vi "PI_GCS2_All_VIs.vi"   [LabVIEW 2026]
doc: "This VI contains all high level and low level VIs valid for PI GCS2 devices. \nSee diagram for a survey of all PI GCS2 high level and low level VIs. \nMenu / Browse / Show VI Hierarchy will show the file paths of the VIs. \nGlobal Variables are shown as Control as well as Indicator."
uses:
  Low Level/Communication/Global1.vi
  Low Level/GeneralCommands/Controller names.ctl
  Low Level/Communication/Available DLL interfaces.ctl
  Low Level/Communication/Available DLLs.ctl
  Low Level/Communication/Available interfaces.ctl
  Low Level/Communication/Termination character.ctl
  Low Level/GeneralCommands/Global2 (Array).vi
  Low Level/Communication/Global DaisyChain.vi
  Low Level/Support/HasCommandArray.vi
  Low Level/Support/GCSArray_regex_selector.ctl
  Low Level/Communication/Syntax.ctl
  Low Level/GeneralCommands/CommandInfo.ctl
  Low Level/GeneralCommands/MemoryType.ctl
  Low Level/GeneralCommands/Parameter Set.ctl
  Low Level/GeneralCommands/ParameterInfoSet.ctl
  Low Level/GeneralCommands/UnitDescription.ctl
  Low Level/SpecialCommand/UserCommandLevel.ctl
  Low Level/Communication/Configuration Setup State.ctl
  Low Level/GeneralCommands/HardwareInfo.ctl
  Low Level/GeneralCommands/DynamicHardwareInfo.ctl
  Low Level/GeneralCommands/FirmwareInfo.ctl
  Low Level/SpecialCommand/RecorderStatus.ctl
  Low Level/SpecialCommand/RecorderTraceConfiguration.ctl
  Low Level/SpecialCommand/RecorderTriggerConfiguration.ctl
  Low Level/SpecialCommand/DriveStateMachine.ctl
  Low Level/SpecialCommand/ModeOfOperation.ctl
  Low Level/GeneralCommands/AxisStatus.ctl
  Low Level/GeneralCommands/SystemStatus.ctl
  Low Level/GeneralCommands/Status.ctl
panel:
  # "PI GCS2 LabVIEW driver set"
  # "This VI contains all high level and low level VIs valid for PI GCS2 devices. See diagram for a survey of all PI GCS2 high level and low level VIs. Menu / Browse / Show VI Hierarchy will show the file paths of the VIs. Global Variables are shown as Control as well as Indicator."
types:
  T1 = typedef "Status.ctl" = cluster{"Element":string, "Status bits":bool[]}
  T2 = typedef "SystemStatus.ctl" = cluster{"Element":string, "Command Error":bool, "Critical Error":bool, "Information":bool, "Warning":bool}
  T3 = typedef "AxisStatus.ctl" = cluster{"Element":string, "Error":bool, "EAX?":bool, "Drive State Machine":T4, "Mode of Operation":T5, "OL/CL control active?":bool, "ONT?":bool, "In Motion":bool, "FRF?":bool, "IPR":bool, "Plim":bool, "Nlim":bool}
  T4 = typedef "DriveStateMachine.ctl" = u16
  T5 = typedef "ModeOfOperation.ctl" = enum16{"Open", "Open-Loop Position", "Closed-Loop Position", "Open-Loop Velocity", "Closed-Loop Velocity", "Open-Loop Force", "Closed-Loop Force", "Step Operation"}
  T6 = typedef "RecorderTriggerConfiguration.ctl" = cluster{"RecorderID":string, "RecorderTrigger":string, "AxisID":string, "Recurring":string}
  T7 = typedef "RecorderTraceConfiguration.ctl" = cluster{"RecorderID":string, "TraceID":i32, "Container Unit":string, "Function Unit":string, "ParameterID":i32}
  T8 = typedef "RecorderStatus.ctl" = enum16{"RUN", "CFG", "WAIT"}
  T9 = typedef "FirmwareInfo.ctl" = cluster{"Container Unit":string, "Function Unit":string, "ID":string, "Mathccode":string, "Version":string, "Date":string, "Compatibility":string, "Description":string}
  T10 = typedef "DynamicHardwareInfo.ctl" = cluster{"Property":string, "Type":string, "Value":string}
  T11 = typedef "HardwareInfo.ctl" = cluster{"Matchcode":string, "Version":string, "Serial Number":string, "Date":string, "Dynamic Hardware":cluster{"Property":string, "Type":string, "Value":string}[], "Firmware":cluster{"Container Unit":string, "Function Unit":string, "ID":string, "Mathccode":string, "Version":string, "Date":string, "Compatibility":string, "Description":string}[]}
  T12 = typedef "Configuration Setup State.ctl" = enum16{"Do nothing", "Initialize indicators", "Select Connection", "TCP/IP Connection", "RS232 Connection", "USB Connection", "Board Connection", "DaisyChain Connection", "Open Interface", "Read IDs", "Prepare referencing", "Reference", "Servo", "Query Status", "Misc", "WaveGenerator", "Control Mode", "Enable Axes", "Translate Error", "Hexapod", "Piezo"}
  T13 = typedef "UserCommandLevel.ctl" = enum16{"User", "Expert", "PI Staff", "FW Developer"}
  T14 = typedef "UnitDescription.ctl" = cluster{"Container Unit":string, "Function Unit":string, "Description":string}
  T15 = typedef "ParameterInfoSet.ctl" = cluster{"Container Unit":string, "Function Unit":string, "Parameter ID":string, "DataType":string, "Dimension":string, "Read UCL":string, "Write UCL":string, "Min Value":string, "Max Value":string, "Parameter Type":string, "Description":string}
  T16 = typedef "Parameter Set.ctl" = cluster{"Memory Type":T17, "Container Unit":string, "Function Unit":string, "Parameter ID":string, "Parameter Value":string}
  T17 = typedef "MemoryType.ctl" = enum16{"<No Setting>", "RAM", "FLASH", "TMP"}
  T18 = typedef "CommandInfo.ctl" = cluster{"Command":string, "Command Signatur":string, "Description":string}
  T19 = typedef "GCSArray_regex_selector.ctl" = enum16{"GCS_ARRAY Block Full", "GCS_ARRAY Block ID", "GCS_ARRAY Block Header", "GCS_ARRAY Block Data", "GCS_ARRAY Identifier", "GCS_ARRAY Remark", "GCS_ARRAY Version", "GCS_ARRAY Dimension", "GCS_ARRAY Type", "GCS_ARRAY Separator", "GCS_ARRAY NData", "GCS_ARRAY NData%", "GCS_ARRAY NData% Keyword", "GCS_ARRAY Name%", "GCS_ARRAY Name% Keyword", "GCS_ARRAY Start%", "GCS_ARRAY Start% Keyword", "GCS_ARRAY End%", "GCS_ARRAY End% Keyword", "GCS_ARRAY Delta%", "GCS_ARRAY Delta% Keword", "GCS_ARRAY Sample Time", "GCS_ARRAY Unit of transmitted value%", "GCS_ARRAY Trans_Unit% Keyword", "GCS_ARRAY Trans_Unit% = RAW Keyword", "GCS_ARRAY Unit of displayed value%", "GCS_ARRAY Disp_Unit% Keyword", "GCS_ARRAY Nominator%", "GCS_ARRAY Ratio_Nom% Keyword", "GCS_ARRAY Denominator%", "GCS_ARRAY Ratio_Denom% Keyword", "GCS_ARRAY End of Header", "GCS_ARRAY Empty line of Header"}
  T20 = typedef "Syntax.ctl" = enum16{"GCS 1.0", "GCS 2.0", "GCS 3.0"}
  T21 = typedef "Termination character.ctl" = enum16{"LF", "CR", "LFCR", "CRLF"}
  T22 = typedef "Available interfaces.ctl" = u16
  T23 = typedef "Available DLLs.ctl" = u16
  T24 = typedef "Available DLL interfaces.ctl" = u16
  T25 = typedef "Controller names.ctl" = enum16{"None", "Analog", "C-702", "C-413", "C-414", "C-843", "C-843.PM", "C-844", "C-848", "C-865", "C-866", "C-867", "C-877", "C-880", "C-884", "C-885", "C-886", "C-887", "C-891", "E-135", "E-516", "E-517", "E-518", "E-709", "E-710", "E-712", "E-725", "E-727", "E-753", "E-754", "E-755", "E-761", "E-816", "E-861", "E-870", "E-871", "E-872", "E-873", "E-874", "F-206", "HydraPollux", "M-840", "M-850", "M-8X0", "Mercury", "Mercury_GCS", "PI_GCS2"}
  T26 = cluster{"No. of devices":i32, "Port ID":i32, "Devices":string[], "Description":string}[]
  T27 = cluster{"Conn. axes":string[], "Controller name":T25}[]
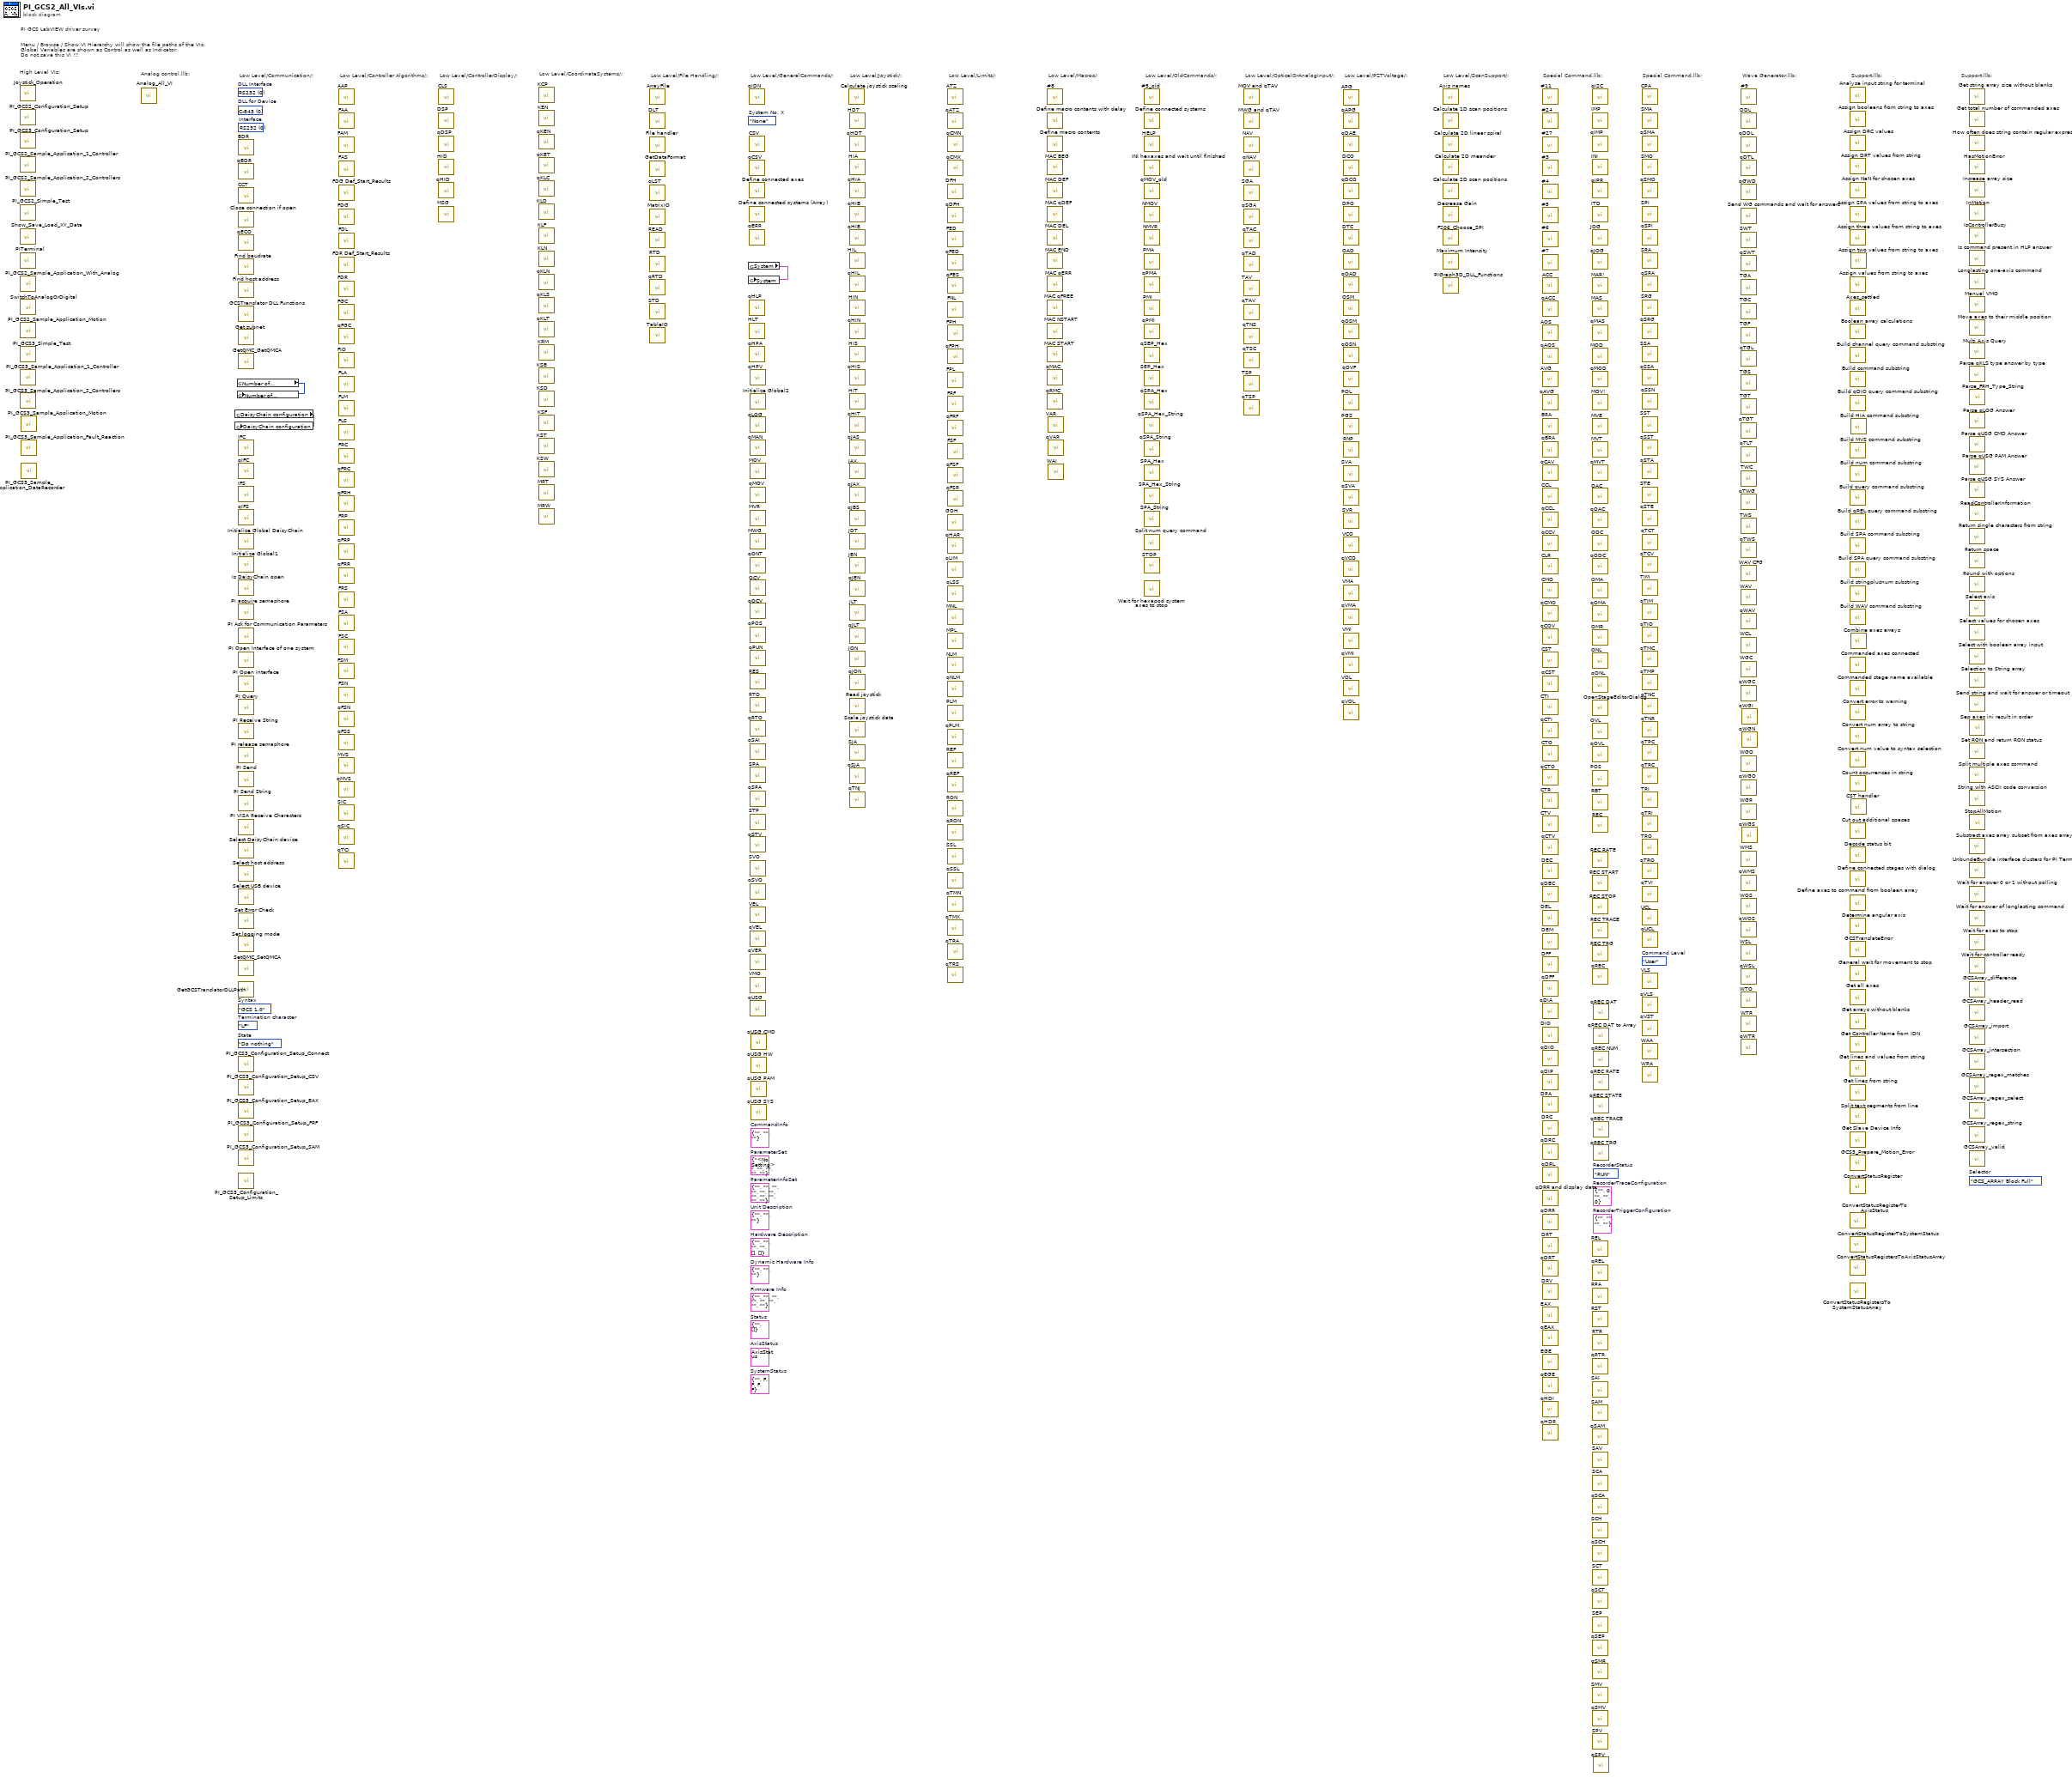
[diagram p0: block diagram]
diagram:
  (unwired) T1 {"Element"="", "Status bits"=[]}  # Status
  (unwired) T2 {"Element"="", "Command Error"=FALSE, "Critical Error"=FALSE, "Information"=FALSE, "Warning"=FALSE}  # SystemStatus
  (unwired) T3 {"Element"="", "Error"=FALSE, "EAX?"=FALSE, "Drive State Machine"=0, "Mode of Operation"=enum."Open", "OL/CL control active?"=FALSE, "ONT?"=FALSE, "In Motion"=FALSE, "FRF?"=FALSE, "IPR"=FALSE, "Plim"=FALSE, "Nlim"=FALSE}  # AxisStatus
  (unwired) T6 {"RecorderID"="", "RecorderTrigger"="", "AxisID"="", "Recurring"=""}  # RecorderTriggerConfiguration
  (unwired) T7 {"RecorderID"="", "TraceID"=0, "Container Unit"="", "Function Unit"="", "ParameterID"=0}  # RecorderTraceConfiguration
  (unwired) RecorderStatus."RUN"  # RecorderStatus
  (unwired) T9 {"Container Unit"="", "Function Unit"="", "ID"="", "Mathccode"="", "Version"="", "Date"="", "Compatibility"="", "Description"=""}  # Firmware Info
  (unwired) T10 {"Property"="", "Type"="", "Value"=""}  # Dynamic Hardware Info
  (unwired) T11 {"Matchcode"="", "Version"="", "Serial Number"="", "Date"="", "Dynamic Hardware"=[], "Firmware"=[]}  # Hardware Description
  (unwired) Configuration_Setup_State."Do nothing"  # State
  (unwired) UserCommandLevel."User"  # Command Level
  (unwired) T14 {"Container Unit"="", "Function Unit"="", "Description"=""}  # Unit Description
  (unwired) T15 {"Container Unit"="", "Function Unit"="", "Parameter ID"="", "DataType"="", "Dimension"="", "Read UCL"="", "Write UCL"="", "Min Value"="", "Max Value"="", "Parameter Type"="", "Description"=""}  # ParameterInfoSet
  (unwired) T16 {"Memory Type"=enum."<No Setting>", "Container Unit"="", "Function Unit"="", "Parameter ID"="", "Parameter Value"=""}  # ParameterSet
  (unwired) T18 {"Command"="", "Command Signatur"="", "Description"=""}  # CommandInfo
  (unwired) GCSArray_regex_selector."GCS_ARRAY Block Full"  # Selector
  (unwired) Syntax."GCS 1.0"  # Syntax
  (unwired) Termination_character."LF"  # Termination character
  (unwired) T22 0 items=["RS232", "GPIB", "DLL", "TCP-IP"]  # Interface
  (unwired) T23 0 items=["C-843", "C-844", "E-710", "C-843.PM", "C-865", "E-761", "Mercury", "E-755", "E-753", "C-866", "E-712", "E-725", "E-861", "C-867", "E-517", "E-816", "E-709", "PI_GCS2_DLL"]  # DLL for Device
  (unwired) T24 0 items=["RS232", "GPIB", "Board", "TCP-IP", "USB", "RS232_DC", "USB_DC"]  # DLL Interface
  (unwired) Controller_names."None"  # System No. X
  # "Low Level/CoordinateSystems/:"
  # "High Level VIs:"
  # "Analog control.llb:"
  # "Support.llb:"
  # "Wave Generator.llb:"
  # "Special Command.llb:"
  # "Support.llb:"
  # "Special Command.llb:"
  # "Low Level/ScanSupport/:"
  # "Low Level/PZTVoltage/:"
  # "Low Level/OpticalOrAnalogInput/:"
  # "Low Level/OldCommands/:"
  # "Low Level/Macros/:"
  # "Low Level/Limits/:"
  # "Low Level/Joystick/:"
  # "Low Level/GeneralCommands/:"
  # "Low Level/File Handling/:"
  # "Low Level/ControllerDisplay/:"
  # "Low Level/Controller Algorithms/:"
  # "Menu / Browse / Show VI Hierarchy will show the file paths of the VIs. \nGlobal Variables are shown as Control as well as Indicator.\nDo not save this VI !!!"
  # "PI GCS LabVIEW driver survey"
  # "Low Level/Communication/:"
  n1 = call "Joystick_Operation.vi"() -> ()  [unwired: 15 in, 5 out]
  n2 = call "PI_GCS2_Configuration_Setup.vi"() -> ()  [unwired: 8 in, 12 out]
  n3 = call "PI_GCS3_Configuration_Setup.vi"() -> ()  [unwired: 14 in, 6 out]
  n4 = call "PI_GCS2_Sample_Application_1_Controller.vi"() -> ()  [unwired: 1 out]
  n5 = call "PI_GCS2_Sample_Application_2_Controllers.vi"() -> ()  [unwired: 1 out]
  n6 = call "PI_GCS2_Simple_Test.vi"() -> ()  [unwired: 20 out]
  n7 = call "Show_Save_Load_XY_Data.vi"() -> ()  [unwired: 7 in, 13 out]
  n8 = call "PITerminal.vi"() -> ()  [unwired: 2 in, 18 out]
  n9 = call "PI_GCS2_Sample_Application_With_Analog.vi"() -> ()  [unwired: 1 out]
  n10 = call "SwitchToAnalogOrDigital.vi"() -> ()  [unwired: 9 in, 11 out]
  n11 = call "PI_GCS2_Sample_Application_Motion.vi"() -> ()  [unwired: 1 in]
  n12 = call "PI_GCS3_Simple_Test.vi"() -> ()  [unwired: 20 in]
  n13 = call "PI_GCS3_Sample_Application_1_Controller.vi"() -> ()  [unwired: 1 in]
  n14 = call "PI_GCS3_Sample_Application_2_Controllers.vi"() -> ()  [unwired: 1 in]
  n15 = call "PI_GCS3_Sample_Application_Motion.vi"() -> ()  [unwired: 1 in]
  n16 = call "PI_GCS3_Sample_Application_Fault_Reaction.vi"() -> ()  [unwired: 20 in]
  n17 = call "PI_GCS3_Sample_Application_DataRecorder.vi"() -> ()  [unwired: 20 in]
  n18 = call "Analog_All_VI.vi"() -> ()  [unwired: 12 out]
  n19 = global read "Global DaisyChain.vi" "DaisyChain configuration"() -> (w1:T26)
  n20 = global write "Global DaisyChain.vi" "DaisyChain configuration"(w1) -> ()
  n21 = global read "Global1.vi" "Number of\nsystems"() -> (w3:i32)
  n22 = global write "Global1.vi" "Number of\nsystems"(w3) -> ()
  n23 = call "BDR.vi"() -> ()  [unwired: 4 in, 16 out]
  n24 = call "qBDR.vi"() -> ()  [unwired: 2 in, 18 out]
  n25 = call "CCT.vi"() -> ()  [unwired: 3 in, 17 out]
  n26 = call "Close connection if open.vi"() -> ()  [unwired: 3 in, 17 out]
  n27 = call "qECO.vi"() -> ()  [unwired: 3 in, 17 out]
  n28 = call "Find baudrate.vi"() -> ()  [unwired: 10 in, 10 out]
  n29 = call "Find host address.vi"() -> ()  [unwired: 6 in, 14 out]
  n30 = call "GCSTranslator DLL Functions.vi"() -> ()  [unwired: 7 in, 13 out]
  n31 = call "Get subnet.vi"() -> ()  [unwired: 20 out]
  n32 = call "GetQMC_GetQMCA.vi"() -> ()  [unwired: 6 in, 14 out]
  n33 = call "IFC.vi"() -> ()  [unwired: 4 in, 16 out]
  n34 = call "qIFC.vi"() -> ()  [unwired: 4 in, 16 out]
  n35 = call "IFS.vi"() -> ()  [unwired: 5 in, 15 out]
  n36 = call "qIFS.vi"() -> ()  [unwired: 4 in, 16 out]
  n37 = call "Initialize Global DaisyChain.vi"() -> ()  [unwired: 2 in, 18 out]
  n38 = call "Initialize Global1.vi"() -> ()  [unwired: 2 in, 18 out]
  n39 = call "Is DaisyChain open.vi"() -> ()  [unwired: 2 in, 18 out]
  n40 = call "PI acquire semaphore.vi"() -> ()  [unwired: 2 in, 18 out]
  n41 = call "PI Ask for Communication Parameters.vi"() -> ()  [unwired: 20 out]
  n42 = call "PI Open Interface of one system.vi"() -> ()  [unwired: 12 in, 8 out]
  n43 = call "PI Open Interface.vi"() -> ()  [unwired: 12 in, 8 out]
  n44 = call "PI Query.vi"() -> ()  [unwired: 7 in, 13 out]
  n45 = call "PI Receive String.vi"() -> ()  [unwired: 3 in, 17 out]
  n46 = call "PI release semaphore.vi"() -> ()  [unwired: 4 in, 16 out]
  n47 = call "PI Send.vi"() -> ()  [unwired: 6 in, 14 out]
  n48 = call "PI Send String.vi"() -> ()  [unwired: 4 in, 16 out]
  n49 = call "PI VISA Receive Characters.vi"() -> ()  [unwired: 3 in, 17 out]
  n50 = call "Select DaisyChain device.vi"() -> ()  [unwired: 9 in, 11 out]
  n51 = call "Select host address.vi"() -> ()  [unwired: 6 in, 14 out]
  n52 = call "Select USB device.vi"() -> ()  [unwired: 5 in, 15 out]
  n53 = call "Set Error Check.vi"() -> ()  [unwired: 2 in, 10 out]
  n54 = call "Set logging mode.vi"() -> ()  [unwired: 4 in, 16 out]
  n55 = call "SetQMC_SetQMCA.vi"() -> ()  [unwired: 8 in, 12 out]
  n56 = call "GetGCSTranslatorDLLPath.vi"() -> ()  [unwired: 1 in, 1 out]
  n57 = call "PI_GCS3_Configuration_Setup_Connect.vi"() -> ()  [unwired: 19 in, 1 out]
  n58 = call "PI_GCS3_Configuration_Setup_CSV.vi"() -> ()  [unwired: 19 in, 1 out]
  n59 = call "PI_GCS3_Configuration_Setup_EAX.vi"() -> ()  [unwired: 19 in, 1 out]
  n60 = call "PI_GCS3_Configuration_Setup_FRF.vi"() -> ()  [unwired: 19 in, 1 out]
  n61 = call "PI_GCS3_Configuration_Setup_SAM.vi"() -> ()  [unwired: 19 in, 1 out]
  n62 = call "PI_GCS3_Configuration_Setup_Limits.vi"() -> ()  [unwired: 17 in, 3 out]
  n63 = call "AAP.vi"() -> ()  [unwired: 12 in, 8 out]
  n64 = call "FAA.vi"() -> ()  [unwired: 11 in, 9 out]
  n65 = call "FAM.vi"() -> ()  [unwired: 11 in, 9 out]
  n66 = call "FAS.vi"() -> ()  [unwired: 11 in, 9 out]
  n67 = call "FDG Def_Start_Results.vi"() -> ()  [unwired: 12 in, 8 out]
  n68 = call "FDG.vi"() -> ()  [unwired: 12 in, 8 out]
  n69 = call "FDL.vi"() -> ()  [unwired: 19 in, 1 out]
  n70 = call "FDR Def_Start_Results.vi"() -> ()  [unwired: 12 in, 8 out]
  n71 = call "FDR.vi"() -> ()  [unwired: 14 in, 6 out]
  n72 = call "FGC.vi"() -> ()  [unwired: 7 in, 13 out]
  n73 = call "qFGC.vi"() -> ()  [unwired: 4 in, 16 out]
  n74 = call "FIO.vi"() -> ()  [unwired: 13 in, 7 out]
  n75 = call "FLA.vi"() -> ()  [unwired: 13 in, 7 out]
  n76 = call "FLM.vi"() -> ()  [unwired: 13 in, 7 out]
  n77 = call "FLS.vi"() -> ()  [unwired: 13 in, 7 out]
  n78 = call "FRC.vi"() -> ()  [unwired: 5 in, 15 out]
  n79 = call "qFRC.vi"() -> ()  [unwired: 4 in, 16 out]
  n80 = call "qFRH.vi"() -> ()  [unwired: 2 in, 18 out]
  n81 = call "FRP.vi"() -> ()  [unwired: 4 in, 16 out]
  n82 = call "qFRP.vi"() -> ()  [unwired: 4 in, 16 out]
  n83 = call "qFRR.vi"() -> ()  [unwired: 6 in, 14 out]
  n84 = call "FRS.vi"() -> ()  [unwired: 3 in, 17 out]
  n85 = call "FSA.vi"() -> ()  [unwired: 13 in, 7 out]
  n86 = call "FSC.vi"() -> ()  [unwired: 12 in, 8 out]
  n87 = call "FSM.vi"() -> ()  [unwired: 12 in, 8 out]
  n88 = call "FSN.vi"() -> ()  [unwired: 13 in, 7 out]
  n89 = call "qFSN.vi"() -> ()  [unwired: 3 in, 17 out]
  n90 = call "qFSS.vi"() -> ()  [unwired: 2 in, 18 out]
  n91 = call "MVS.vi"() -> ()  [unwired: 8 in, 12 out]
  n92 = call "qMVS.vi"() -> ()  [unwired: 5 in, 15 out]
  n93 = call "SIC.vi"() -> ()  [unwired: 6 in, 14 out]
  n94 = call "qSIC.vi"() -> ()  [unwired: 4 in, 16 out]
  n95 = call "qTCI.vi"() -> ()  [unwired: 3 in, 17 out]
  n96 = call "CLS.vi"() -> ()  [unwired: 2 in, 18 out]
  n97 = call "DSP.vi"() -> ()  [unwired: 5 in, 15 out]
  n98 = call "qDSP.vi"() -> ()  [unwired: 3 in, 17 out]
  n99 = call "HID.vi"() -> ()  [unwired: 5 in, 15 out]
  n100 = call "qHID.vi"() -> ()  [unwired: 3 in, 17 out]
  n101 = call "MSG.vi"() -> ()  [unwired: 3 in, 17 out]
  n102 = call "KCP.vi"() -> ()  [unwired: 4 in, 16 out]
  n103 = call "KEN.vi"() -> ()  [unwired: 3 in, 17 out]
  n104 = call "qKEN.vi"() -> ()  [unwired: 3 in, 17 out]
  n105 = call "qKET.vi"() -> ()  [unwired: 3 in, 17 out]
  n106 = call "qKLC.vi"() -> ()  [unwired: 6 in, 14 out]
  n107 = call "KLD.vi"() -> ()  [unwired: 6 in, 14 out]
  n108 = call "KLF.vi"() -> ()  [unwired: 3 in, 17 out]
  n109 = call "KLN.vi"() -> ()  [unwired: 4 in, 16 out]
  n110 = call "qKLN.vi"() -> ()  [unwired: 3 in, 17 out]
  n111 = call "qKLS.vi"() -> ()  [unwired: 5 in, 15 out]
  n112 = call "qKLT.vi"() -> ()  [unwired: 4 in, 16 out]
  n113 = call "KRM.vi"() -> ()  [unwired: 3 in, 17 out]
  n114 = call "KSB.vi"() -> ()  [unwired: 6 in, 14 out]
  n115 = call "KSD.vi"() -> ()  [unwired: 6 in, 14 out]
  n116 = call "KSF.vi"() -> ()  [unwired: 3 in, 17 out]
  n117 = call "KST.vi"() -> ()  [unwired: 6 in, 14 out]
  n118 = call "KSW.vi"() -> ()  [unwired: 6 in, 14 out]
  n119 = call "MRT.vi"() -> ()  [unwired: 5 in, 15 out]
  n120 = call "MRW.vi"() -> ()  [unwired: 5 in, 15 out]
  n121 = call "ArrayFile.vi"() -> ()  [unwired: 20 out]
  n122 = call "DLT.vi"() -> ()  [unwired: 3 in, 17 out]
  n123 = call "File handler.vi"() -> ()  [unwired: 6 in, 14 out]
  n124 = call "GetDataFormat.vi"() -> ()  [unwired: 2 in, 18 out]
  n125 = call "qLST.vi"() -> ()  [unwired: 2 in, 18 out]
  n126 = call "MatrixIO.vi"() -> ()  [unwired: 7 in, 13 out]
  n127 = call "READ.vi"() -> ()  [unwired: 3 in, 17 out]
  n128 = call "RTD.vi"() -> ()  [unwired: 5 in, 15 out]
  n129 = call "qRTD.vi"() -> ()  [unwired: 2 in, 18 out]
  n130 = call "STD.vi"() -> ()  [unwired: 5 in, 15 out]
  n131 = call "TableIO.vi"() -> ()  [unwired: 6 in, 14 out]
  n132 = global read "Global2 (Array).vi" "System"() -> (w2:T27)
  n133 = global write "Global2 (Array).vi" "System"(w2) -> ()
  n134 = call "qIDN.vi"() -> ()  [unwired: 2 in, 18 out]
  n135 = call "CSV.vi"() -> ()  [unwired: 3 in, 17 out]
  n136 = call "qCSV.vi"() -> ()  [unwired: 2 in, 18 out]
  n137 = call "Define connected axes.vi"() -> ()  [unwired: 5 in, 15 out]
  n138 = call "Define connected systems (Array).vi"() -> ()  [unwired: 4 in, 16 out]
  n139 = call "qERR.vi"() -> ()  [unwired: 2 in, 18 out]
  n140 = call "qHLP.vi"() -> ()  [unwired: 2 in, 18 out]
  n141 = call "HLT.vi"() -> ()  [unwired: 5 in, 15 out]
  n142 = call "qHPA.vi"() -> ()  [unwired: 2 in, 18 out]
  n143 = call "qHPV.vi"() -> ()  [unwired: 2 in, 18 out]
  n144 = call "Initialize Global2.vi"() -> ()  [unwired: 2 in, 18 out]
  n145 = call "qLOG.vi"() -> ()  [unwired: 18 in, 2 out]
  n146 = call "qMAN.vi"() -> ()  [unwired: 3 in, 17 out]
  n147 = call "MOV.vi"() -> ()  [unwired: 5 in, 15 out]
  n148 = call "qMOV.vi"() -> ()  [unwired: 5 in, 15 out]
  n149 = call "MVR.vi"() -> ()  [unwired: 5 in, 15 out]
  n150 = call "MWG.vi"() -> ()  [unwired: 5 in, 15 out]
  n151 = call "qONT.vi"() -> ()  [unwired: 5 in, 15 out]
  n152 = call "OCV.vi"() -> ()  [unwired: 19 in, 1 out]
  n153 = call "qOCV.vi"() -> ()  [unwired: 18 in, 2 out]
  n154 = call "qPOS.vi"() -> ()  [unwired: 5 in, 15 out]
  n155 = call "qPUN.vi"() -> ()  [unwired: 5 in, 15 out]
  n156 = call "RES.vi"() -> ()  [unwired: 19 in, 1 out]
  n157 = call "RTO.vi"() -> ()  [unwired: 5 in, 15 out]
  n158 = call "qRTO.vi"() -> ()  [unwired: 5 in, 15 out]
  n159 = call "qSAI.vi"() -> ()  [unwired: 5 in, 15 out]
  n160 = call "SPA.vi"() -> ()  [unwired: 10 in, 10 out]
  n161 = call "qSPA.vi"() -> ()  [unwired: 7 in, 13 out]
  n162 = call "STP.vi"() -> ()  [unwired: 2 in, 18 out]
  n163 = call "qSTV.vi"() -> ()  [unwired: 18 in, 2 out]
  n164 = call "SVO.vi"() -> ()  [unwired: 5 in, 15 out]
  n165 = call "qSVO.vi"() -> ()  [unwired: 5 in, 15 out]
  n166 = call "VEL.vi"() -> ()  [unwired: 6 in, 14 out]
  n167 = call "qVEL.vi"() -> ()  [unwired: 5 in, 15 out]
  n168 = call "qVER.vi"() -> ()  [unwired: 2 in, 18 out]
  n169 = call "VMO.vi"() -> ()  [unwired: 5 in, 15 out]
  n170 = call-poly "qUSG.vi"() -> ()  [unwired: 18 in, 2 out]
  n171 = call "qUSG CMD.vi"() -> ()  [unwired: 18 in, 2 out]
  n172 = call "qUSG HW.vi"() -> ()  [unwired: 18 in, 2 out]
  n173 = call "qUSG PAM.vi"() -> ()  [unwired: 18 in, 2 out]
  n174 = call "qUSG SYS.vi"() -> ()  [unwired: 18 in, 2 out]
  n175 = call "Calculate joystick scaling.vi"() -> ()  [unwired: 6 in, 14 out]
  n176 = call "HDT.vi"() -> ()  [unwired: 5 in, 15 out]
  n177 = call "qHDT.vi"() -> ()  [unwired: 5 in, 15 out]
  n178 = call "HIA.vi"() -> ()  [unwired: 6 in, 14 out]
  n179 = call "qHIA.vi"() -> ()  [unwired: 5 in, 15 out]
  n180 = call "qHIB.vi"() -> ()  [unwired: 5 in, 15 out]
  n181 = call "qHIE.vi"() -> ()  [unwired: 5 in, 15 out]
  n182 = call "HIL.vi"() -> ()  [unwired: 5 in, 15 out]
  n183 = call "qHIL.vi"() -> ()  [unwired: 5 in, 15 out]
  n184 = call "HIN.vi"() -> ()  [unwired: 4 in, 16 out]
  n185 = call "qHIN.vi"() -> ()  [unwired: 5 in, 15 out]
  n186 = call "HIS.vi"() -> ()  [unwired: 6 in, 14 out]
  n187 = call "qHIS.vi"() -> ()  [unwired: 6 in, 14 out]
  n188 = call "HIT.vi"() -> ()  [unwired: 5 in, 15 out]
  n189 = call "qHIT.vi"() -> ()  [unwired: 7 in, 13 out]
  n190 = call "qJAS.vi"() -> ()  [unwired: 5 in, 15 out]
  n191 = call "JAX.vi"() -> ()  [unwired: 5 in, 15 out]
  n192 = call "qJAX.vi"() -> ()  [unwired: 5 in, 15 out]
  n193 = call "qJBS.vi"() -> ()  [unwired: 5 in, 15 out]
  n194 = call "JDT.vi"() -> ()  [unwired: 5 in, 15 out]
  n195 = call "JEN.vi"() -> ()  [unwired: 3 in, 17 out]
  n196 = call "qJEN.vi"() -> ()  [unwired: 2 in, 18 out]
  n197 = call "JLT.vi"() -> ()  [unwired: 7 in, 13 out]
  n198 = call "qJLT.vi"() -> ()  [unwired: 7 in, 13 out]
  n199 = call "JON.vi"() -> ()  [unwired: 4 in, 16 out]
  n200 = call "qJON.vi"() -> ()  [unwired: 4 in, 16 out]
  n201 = call "Read joystick.vi"() -> ()  [unwired: 2 in, 18 out]
  n202 = call "Scale joystick data.vi"() -> ()  [unwired: 8 in, 12 out]
  n203 = call "SJA.vi"() -> ()  [unwired: 4 in, 16 out]
  n204 = call "qSJA.vi"() -> ()  [unwired: 3 in, 17 out]
  n205 = call "qTNJ.vi"() -> ()  [unwired: 2 in, 18 out]
  n206 = call "ATZ.vi"() -> ()  [unwired: 6 in, 14 out]
  n207 = call "qATZ.vi"() -> ()  [unwired: 5 in, 15 out]
  n208 = call "DFH.vi"() -> ()  [unwired: 5 in, 15 out]
  n209 = call "qDFH.vi"() -> ()  [unwired: 5 in, 15 out]
  n210 = call "FED.vi"() -> ()  [unwired: 5 in, 15 out]
  n211 = call "qFED.vi"() -> ()  [unwired: 5 in, 15 out]
  n212 = call "qFES.vi"() -> ()  [unwired: 5 in, 15 out]
  n213 = call "FNL.vi"() -> ()  [unwired: 5 in, 15 out]
  n214 = call "FPL.vi"() -> ()  [unwired: 5 in, 15 out]
  n215 = call "FRF.vi"() -> ()  [unwired: 5 in, 15 out]
  n216 = call "qFRF.vi"() -> ()  [unwired: 5 in, 15 out]
  n217 = call "GOH.vi"() -> ()  [unwired: 5 in, 15 out]
  n218 = call "qHAR.vi"() -> ()  [unwired: 5 in, 15 out]
  n219 = call "qLIM.vi"() -> ()  [unwired: 5 in, 15 out]
  n220 = call "qLSS.vi"() -> ()  [unwired: 5 in, 15 out]
  n221 = call "MNL.vi"() -> ()  [unwired: 5 in, 15 out]
  n222 = call "MPL.vi"() -> ()  [unwired: 5 in, 15 out]
  n223 = call "NLM.vi"() -> ()  [unwired: 5 in, 15 out]
  n224 = call "qNLM.vi"() -> ()  [unwired: 5 in, 15 out]
  n225 = call "PLM.vi"() -> ()  [unwired: 5 in, 15 out]
  n226 = call "qPLM.vi"() -> ()  [unwired: 5 in, 15 out]
  n227 = call "REF.vi"() -> ()  [unwired: 5 in, 15 out]
  n228 = call "qREF.vi"() -> ()  [unwired: 5 in, 15 out]
  n229 = call "RON.vi"() -> ()  [unwired: 5 in, 15 out]
  n230 = call "qRON.vi"() -> ()  [unwired: 5 in, 15 out]
  n231 = call "SSL.vi"() -> ()  [unwired: 5 in, 15 out]
  n232 = call "qSSL.vi"() -> ()  [unwired: 5 in, 15 out]
  n233 = call "qTMN.vi"() -> ()  [unwired: 5 in, 15 out]
  n234 = call "qTMX.vi"() -> ()  [unwired: 5 in, 15 out]
  n235 = call "qTRS.vi"() -> ()  [unwired: 5 in, 15 out]
  n236 = call "qCMN.vi"() -> ()  [unwired: 5 in, 15 out]
  n237 = call "qCMX.vi"() -> ()  [unwired: 5 in, 15 out]
  n238 = call "FPH.vi"() -> ()  [unwired: 5 in, 15 out]
  n239 = call "qFPH.vi"() -> ()  [unwired: 5 in, 15 out]
  n240 = call "FSF.vi"() -> ()  [unwired: 8 in, 12 out]
  n241 = call "qFSF.vi"() -> ()  [unwired: 5 in, 15 out]
  n242 = call "qFSR.vi"() -> ()  [unwired: 4 in, 16 out]
  n243 = call "qTRA.vi"() -> ()  [unwired: 5 in, 15 out]
  n244 = call "#8.vi"() -> ()  [unwired: 2 in, 18 out]
  n245 = call "Define macro contents with delay.vi"() -> ()  [unwired: 4 in, 16 out]
  n246 = call "Define macro contents.vi"() -> ()  [unwired: 3 in, 17 out]
  n247 = call "MAC BEG.vi"() -> ()  [unwired: 3 in, 17 out]
  n248 = call "MAC DEF.vi"() -> ()  [unwired: 3 in, 17 out]
  n249 = call "MAC qDEF.vi"() -> ()  [unwired: 2 in, 18 out]
  n250 = call "MAC DEL.vi"() -> ()  [unwired: 4 in, 16 out]
  n251 = call "MAC END.vi"() -> ()  [unwired: 2 in, 18 out]
  n252 = call "MAC qERR.vi"() -> ()  [unwired: 2 in, 18 out]
  n253 = call "MAC qFREE.vi"() -> ()  [unwired: 2 in, 18 out]
  n254 = call "MAC NSTART.vi"() -> ()  [unwired: 5 in, 15 out]
  n255 = call "MAC START.vi"() -> ()  [unwired: 4 in, 16 out]
  n256 = call "qMAC.vi"() -> ()  [unwired: 4 in, 16 out]
  n257 = call "qRMC.vi"() -> ()  [unwired: 2 in, 18 out]
  n258 = call "VAR.vi"() -> ()  [unwired: 4 in, 16 out]
  n259 = call "qVAR.vi"() -> ()  [unwired: 4 in, 16 out]
  n260 = call "WAI.vi"() -> ()  [unwired: 5 in, 15 out]
  n261 = call "#5_old.vi"() -> ()  [unwired: 2 in, 18 out]
  n262 = call "Define connected systems.vi"() -> ()  [unwired: 4 in, 16 out]
  n263 = call "HELP.vi"() -> ()  [unwired: 2 in, 18 out]
  n264 = call "INI hexaxes and wait until finished.vi"() -> ()  [unwired: 6 in, 14 out]
  n265 = call "qMOV_old.vi"() -> ()  [unwired: 3 in, 17 out]
  n266 = call "NMOV.vi"() -> ()  [unwired: 5 in, 15 out]
  n267 = call "NMVR.vi"() -> ()  [unwired: 5 in, 15 out]
  n268 = call "PMA.vi"() -> ()  [unwired: 5 in, 15 out]
  n269 = call "qPMA.vi"() -> ()  [unwired: 5 in, 15 out]
  n270 = call "PMI.vi"() -> ()  [unwired: 5 in, 15 out]
  n271 = call "qPMI.vi"() -> ()  [unwired: 5 in, 15 out]
  n272 = call "qSEP_Hex.vi"() -> ()  [unwired: 5 in, 15 out]
  n273 = call "SEP_Hex.vi"() -> ()  [unwired: 6 in, 14 out]
  n274 = call "qSPA_Hex.vi"() -> ()  [unwired: 5 in, 15 out]
  n275 = call "qSPA_Hex_String.vi"() -> ()  [unwired: 5 in, 15 out]
  n276 = call "qSPA_String.vi"() -> ()  [unwired: 4 in, 16 out]
  n277 = call "SPA_Hex.vi"() -> ()  [unwired: 6 in, 14 out]
  n278 = call "SPA_Hex_String.vi"() -> ()  [unwired: 5 in, 15 out]
  n279 = call "SPA_String.vi"() -> ()  [unwired: 5 in, 15 out]
  n280 = call "Split num query command.vi"() -> ()  [unwired: 4 in, 16 out]
  n281 = call "STOP.vi"() -> ()  [unwired: 2 in, 18 out]
  n282 = call "Wait for hexapod system axes to stop.vi"() -> ()  [unwired: 5 in, 15 out]
  n283 = call "MOV and qTAV.vi"() -> ()  [unwired: 9 in, 11 out]
  n284 = call "MWG and qTAV.vi"() -> ()  [unwired: 9 in, 11 out]
  n285 = call "NAV.vi"() -> ()  [unwired: 4 in, 16 out]
  n286 = call "qNAV.vi"() -> ()  [unwired: 3 in, 17 out]
  n287 = call "SGA.vi"() -> ()  [unwired: 4 in, 16 out]
  n288 = call "qSGA.vi"() -> ()  [unwired: 3 in, 17 out]
  n289 = call "qTAC.vi"() -> ()  [unwired: 2 in, 18 out]
  n290 = call "qTAD.vi"() -> ()  [unwired: 5 in, 15 out]
  n291 = call "TAV.vi"() -> ()  [unwired: 7 in, 13 out]
  n292 = call "qTAV.vi"() -> ()  [unwired: 4 in, 16 out]
  n293 = call "qTNS.vi"() -> ()  [unwired: 5 in, 15 out]
  n294 = call "qTSC.vi"() -> ()  [unwired: 2 in, 18 out]
  n295 = call "TSP.vi"() -> ()  [unwired: 5 in, 15 out]
  n296 = call "qTSP.vi"() -> ()  [unwired: 5 in, 15 out]
  n297 = call "APG.vi"() -> ()  [unwired: 5 in, 15 out]
  n298 = call "qAPG.vi"() -> ()  [unwired: 5 in, 15 out]
  n299 = call "qDAE.vi"() -> ()  [unwired: 5 in, 15 out]
  n300 = call "DCO.vi"() -> ()  [unwired: 4 in, 16 out]
  n301 = call "qDCO.vi"() -> ()  [unwired: 5 in, 15 out]
  n302 = call "DPO.vi"() -> ()  [unwired: 5 in, 15 out]
  n303 = call "DTC.vi"() -> ()  [unwired: 4 in, 16 out]
  n304 = call "OAD.vi"() -> ()  [unwired: 5 in, 15 out]
  n305 = call "qOAD.vi"() -> ()  [unwired: 5 in, 15 out]
  n306 = call "OSM.vi"() -> ()  [unwired: 5 in, 15 out]
  n307 = call "qOSM.vi"() -> ()  [unwired: 5 in, 15 out]
  n308 = call "qOSN.vi"() -> ()  [unwired: 5 in, 15 out]
  n309 = call "qOVF.vi"() -> ()  [unwired: 5 in, 15 out]
  n310 = call "POL.vi"() -> ()  [unwired: 4 in, 16 out]
  n311 = call "PGS.vi"() -> ()  [unwired: 5 in, 15 out]
  n312 = call "RNP.vi"() -> ()  [unwired: 6 in, 14 out]
  n313 = call "SVA.vi"() -> ()  [unwired: 5 in, 15 out]
  n314 = call "qSVA.vi"() -> ()  [unwired: 5 in, 15 out]
  n315 = call "SVR.vi"() -> ()  [unwired: 5 in, 15 out]
  n316 = call "VCO.vi"() -> ()  [unwired: 4 in, 16 out]
  n317 = call "qVCO.vi"() -> ()  [unwired: 5 in, 15 out]
  n318 = call "VMA.vi"() -> ()  [unwired: 5 in, 15 out]
  n319 = call "qVMA.vi"() -> ()  [unwired: 5 in, 15 out]
  n320 = call "VMI.vi"() -> ()  [unwired: 5 in, 15 out]
  n321 = call "qVMI.vi"() -> ()  [unwired: 5 in, 15 out]
  n322 = call "VOL.vi"() -> ()  [unwired: 5 in, 15 out]
  n323 = call "qVOL.vi"() -> ()  [unwired: 5 in, 15 out]
  n324 = call "Axis names.vi"() -> ()  [unwired: 1 in, 19 out]
  n325 = call "Calculate 1D scan positions.vi"() -> ()  [unwired: 4 in, 16 out]
  n326 = call "Calculate 2D linear spiral.vi"() -> ()  [unwired: 4 in, 16 out]
  n327 = call "Calculate 2D meander.vi"() -> ()  [unwired: 8 in, 12 out]
  n328 = call "Calculate 2D scan positions.vi"() -> ()  [unwired: 7 in, 13 out]
  n329 = call "Decrease Gain.vi"() -> ()  [unwired: 6 in, 14 out]
  n330 = call "F206_Choose_SPI.vi"() -> ()  [unwired: 4 in, 16 out]
  n331 = call "Maximum Intensity.vi"() -> ()  [unwired: 8 in, 12 out]
  n332 = call "PIGraph3D_DLL_Functions.vi"() -> ()  [unwired: 13 in, 7 out]
  n333 = call "#11.vi"() -> ()  [unwired: 2 in, 18 out]
  n334 = call "#24.vi"() -> ()  [unwired: 2 in, 18 out]
  n335 = call "#27.vi"() -> ()  [unwired: 2 in, 18 out]
  n336 = call "#3.vi"() -> ()  [unwired: 2 in, 18 out]
  n337 = call "#4.vi"() -> ()  [unwired: 2 in, 18 out]
  n338 = call "#5.vi"() -> ()  [unwired: 2 in, 18 out]
  n339 = call "#6.vi"() -> ()  [unwired: 2 in, 18 out]
  n340 = call "#7.vi"() -> ()  [unwired: 2 in, 18 out]
  n341 = call "ACC.vi"() -> ()  [unwired: 6 in, 14 out]
  n342 = call "qACC.vi"() -> ()  [unwired: 5 in, 15 out]
  n343 = call "AOS.vi"() -> ()  [unwired: 5 in, 15 out]
  n344 = call "qAOS.vi"() -> ()  [unwired: 5 in, 15 out]
  n345 = call "AVG.vi"() -> ()  [unwired: 3 in, 17 out]
  n346 = call "qAVG.vi"() -> ()  [unwired: 2 in, 18 out]
  n347 = call "BRA.vi"() -> ()  [unwired: 4 in, 16 out]
  n348 = call "qBRA.vi"() -> ()  [unwired: 5 in, 15 out]
  n349 = call "qCAV.vi"() -> ()  [unwired: 5 in, 15 out]
  n350 = call "CCL.vi"() -> ()  [unwired: 4 in, 16 out]
  n351 = call "CLR.vi"() -> ()  [unwired: 5 in, 15 out]
  n352 = call "qCMO.vi"() -> ()  [unwired: 5 in, 15 out]
  n353 = call "qCOV.vi"() -> ()  [unwired: 4 in, 16 out]
  n354 = call "CST.vi"() -> ()  [unwired: 4 in, 16 out]
  n355 = call "qCST.vi"() -> ()  [unwired: 5 in, 15 out]
  n356 = call "CTI.vi"() -> ()  [unwired: 6 in, 14 out]
  n357 = call "qCTI.vi"() -> ()  [unwired: 5 in, 15 out]
  n358 = call "CTO.vi"() -> ()  [unwired: 6 in, 14 out]
  n359 = call "qCTO.vi"() -> ()  [unwired: 5 in, 15 out]
  n360 = call "CTR.vi"() -> ()  [unwired: 5 in, 15 out]
  n361 = call "CTV.vi"() -> ()  [unwired: 5 in, 15 out]
  n362 = call "DEC.vi"() -> ()  [unwired: 6 in, 14 out]
  n363 = call "qDEC.vi"() -> ()  [unwired: 5 in, 15 out]
  n364 = call "DEL.vi"() -> ()  [unwired: 3 in, 17 out]
  n365 = call "DEM.vi"() -> ()  [unwired: 2 in, 18 out]
  n366 = call "DFF.vi"() -> ()  [unwired: 5 in, 15 out]
  n367 = call "qDFF.vi"() -> ()  [unwired: 5 in, 15 out]
  n368 = call "qDIA.vi"() -> ()  [unwired: 4 in, 16 out]
  n369 = call "DIO.vi"() -> ()  [unwired: 6 in, 14 out]
  n370 = call "qDIO.vi"() -> ()  [unwired: 6 in, 14 out]
  n371 = call "qDIP.vi"() -> ()  [unwired: 5 in, 15 out]
  n372 = call "DPA.vi"() -> ()  [unwired: 7 in, 13 out]
  n373 = call "DRC.vi"() -> ()  [unwired: 6 in, 14 out]
  n374 = call "qDRC.vi"() -> ()  [unwired: 4 in, 16 out]
  n375 = call "qDRL.vi"() -> ()  [unwired: 4 in, 16 out]
  n376 = call "qDRR and display data.vi"() -> ()  [unwired: 7 in, 13 out]
  n377 = call "qDRR.vi"() -> ()  [unwired: 8 in, 12 out]
  n378 = call "DRT.vi"() -> ()  [unwired: 5 in, 15 out]
  n379 = call "qDRT.vi"() -> ()  [unwired: 4 in, 16 out]
  n380 = call "DRV.vi"() -> ()  [unwired: 4 in, 16 out]
  n381 = call "EAX.vi"() -> ()  [unwired: 4 in, 16 out]
  n382 = call "EGE.vi"() -> ()  [unwired: 5 in, 15 out]
  n383 = call "qEGE.vi"() -> ()  [unwired: 5 in, 15 out]
  n384 = call "qHDI.vi"() -> ()  [unwired: 2 in, 18 out]
  n385 = call "qHDR.vi"() -> ()  [unwired: 3 in, 17 out]
  n386 = call "qCCL.vi"() -> ()  [unwired: 2 in, 18 out]
  n387 = call "qCCV.vi"() -> ()  [unwired: 5 in, 15 out]
  n388 = call "CMO.vi"() -> ()  [unwired: 4 in, 16 out]
  n389 = call "qCTV.vi"() -> ()  [unwired: 5 in, 15 out]
  n390 = call "qEAX.vi"() -> ()  [unwired: 5 in, 15 out]
  n391 = call "qI2C.vi"() -> ()  [unwired: 2 in, 18 out]
  n392 = call "IMP.vi"() -> ()  [unwired: 5 in, 15 out]
  n393 = call "qIMP.vi"() -> ()  [unwired: 6 in, 14 out]
  n394 = call "INI.vi"() -> ()  [unwired: 5 in, 15 out]
  n395 = call "qIPR.vi"() -> ()  [unwired: 18 in, 2 out]
  n396 = call "ITD.vi"() -> ()  [unwired: 5 in, 15 out]
  n397 = call "JOG.vi"() -> ()  [unwired: 5 in, 15 out]
  n398 = call "qJOG.vi"() -> ()  [unwired: 5 in, 15 out]
  n399 = call "MAR!.vi"() -> ()  [unwired: 5 in, 15 out]
  n400 = call "MAS.vi"() -> ()  [unwired: 4 in, 16 out]
  n401 = call "qMAS.vi"() -> ()  [unwired: 5 in, 15 out]
  n402 = call "MOV!.vi"() -> ()  [unwired: 5 in, 15 out]
  n403 = call "MVE.vi"() -> ()  [unwired: 5 in, 15 out]
  n404 = call "MVT.vi"() -> ()  [unwired: 5 in, 15 out]
  n405 = call "qMVT.vi"() -> ()  [unwired: 5 in, 15 out]
  n406 = call "OAC.vi"() -> ()  [unwired: 6 in, 14 out]
  n407 = call "qOAC.vi"() -> ()  [unwired: 5 in, 15 out]
  n408 = call "ODC.vi"() -> ()  [unwired: 6 in, 14 out]
  n409 = call "qODC.vi"() -> ()  [unwired: 5 in, 15 out]
  n410 = call "OMA.vi"() -> ()  [unwired: 5 in, 15 out]
  n411 = call "qOMA.vi"() -> ()  [unwired: 5 in, 15 out]
  n412 = call "OMR.vi"() -> ()  [unwired: 5 in, 15 out]
  n413 = call "ONL.vi"() -> ()  [unwired: 5 in, 15 out]
  n414 = call "qONL.vi"() -> ()  [unwired: 4 in, 16 out]
  n415 = call "OpenStageEditorDialog.vi"() -> ()  [unwired: 3 in, 17 out]
  n416 = call "OVL.vi"() -> ()  [unwired: 5 in, 15 out]
  n417 = call "qOVL.vi"() -> ()  [unwired: 4 in, 16 out]
  n418 = call "POS.vi"() -> ()  [unwired: 5 in, 15 out]
  n419 = call "RBT.vi"() -> ()  [unwired: 2 in, 18 out]
  n420 = call-poly "REC.vi"() -> ()  [unwired: 19 in, 1 out]
  n421 = call "REL.vi"() -> ()  [unwired: 4 in, 16 out]
  n422 = call "qREL.vi"() -> ()  [unwired: 5 in, 15 out]
  n423 = call "RPA.vi"() -> ()  [unwired: 6 in, 14 out]
  n424 = call "RST.vi"() -> ()  [unwired: 5 in, 15 out]
  n425 = call "RTR.vi"() -> ()  [unwired: 3 in, 17 out]
  n426 = call "qRTR.vi"() -> ()  [unwired: 2 in, 18 out]
  n427 = call "SAI.vi"() -> ()  [unwired: 4 in, 16 out]
  n428 = call "MOD.vi"() -> ()  [unwired: 5 in, 15 out]
  n429 = call "qMOD.vi"() -> ()  [unwired: 5 in, 15 out]
  n430 = call "REC RATE.vi"() -> ()  [unwired: 19 in, 1 out]
  n431 = call "REC START.vi"() -> ()  [unwired: 19 in, 1 out]
  n432 = call "REC STOP.vi"() -> ()  [unwired: 19 in, 1 out]
  n433 = call "REC TRACE.vi"() -> ()  [unwired: 19 in, 1 out]
  n434 = call "REC TRG.vi"() -> ()  [unwired: 19 in, 1 out]
  n435 = call-poly "qREC.vi"() -> ()  [unwired: 18 in, 2 out]
  n436 = call "SAM.vi"() -> ()  [unwired: 19 in, 1 out]
  n437 = call "qSAM.vi"() -> ()  [unwired: 18 in, 2 out]
  n438 = call "SAV.vi"() -> ()  [unwired: 5 in, 15 out]
  n439 = call "SCA.vi"() -> ()  [unwired: 4 in, 16 out]
  n440 = call "qSCA.vi"() -> ()  [unwired: 2 in, 18 out]
  n441 = call "SCH.vi"() -> ()  [unwired: 3 in, 17 out]
  n442 = call "qSCH.vi"() -> ()  [unwired: 2 in, 18 out]
  n443 = call "SCT.vi"() -> ()  [unwired: 3 in, 17 out]
  n444 = call "qSCT.vi"() -> ()  [unwired: 2 in, 18 out]
  n445 = call "SEP.vi"() -> ()  [unwired: 11 in, 9 out]
  n446 = call "qSEP.vi"() -> ()  [unwired: 7 in, 13 out]
  n447 = call "qSMR.vi"() -> ()  [unwired: 18 in, 2 out]
  n448 = call "SMV.vi"() -> ()  [unwired: 19 in, 1 out]
  n449 = call "qSMV.vi"() -> ()  [unwired: 18 in, 2 out]
  n450 = call "SPV.vi"() -> ()  [unwired: 19 in, 1 out]
  n451 = call "qREC DAT.vi"() -> ()  [unwired: 18 in, 2 out]
  n452 = call "qREC DAT to Array.vi"() -> ()  [unwired: 17 in, 3 out]
  n453 = call "qREC NUM.vi"() -> ()  [unwired: 18 in, 2 out]
  n454 = call "qREC RATE.vi"() -> ()  [unwired: 18 in, 2 out]
  n455 = call "qREC STATE.vi"() -> ()  [unwired: 18 in, 2 out]
  n456 = call "qREC TRACE.vi"() -> ()  [unwired: 18 in, 2 out]
  n457 = call "qREC TRG.vi"() -> ()  [unwired: 18 in, 2 out]
  n458 = call "qSPV.vi"() -> ()  [unwired: 18 in, 2 out]
  n459 = call "CPA.vi"() -> ()  [unwired: 19 in, 1 out]
  n460 = call "SMA.vi"() -> ()  [unwired: 4 in, 16 out]
  n461 = call "qSMA.vi"() -> ()  [unwired: 3 in, 17 out]
  n462 = call "SMO.vi"() -> ()  [unwired: 4 in, 16 out]
  n463 = call "qSMO.vi"() -> ()  [unwired: 5 in, 15 out]
  n464 = call "SPI.vi"() -> ()  [unwired: 3 in, 17 out]
  n465 = call "qSPI.vi"() -> ()  [unwired: 2 in, 18 out]
  n466 = call "SRA.vi"() -> ()  [unwired: 5 in, 15 out]
  n467 = call "qSRA.vi"() -> ()  [unwired: 5 in, 15 out]
  n468 = call "SRG.vi"() -> ()  [unwired: 6 in, 14 out]
  n469 = call "qSRG.vi"() -> ()  [unwired: 5 in, 15 out]
  n470 = call "SSA.vi"() -> ()  [unwired: 5 in, 15 out]
  n471 = call "qSSA.vi"() -> ()  [unwired: 5 in, 15 out]
  n472 = call "qSSN.vi"() -> ()  [unwired: 4 in, 16 out]
  n473 = call "SST.vi"() -> ()  [unwired: 5 in, 15 out]
  n474 = call "qSST.vi"() -> ()  [unwired: 5 in, 15 out]
  n475 = call "qSTA.vi"() -> ()  [unwired: 5 in, 15 out]
  n476 = call "STE.vi"() -> ()  [unwired: 6 in, 14 out]
  n477 = call "qSTE.vi"() -> ()  [unwired: 6 in, 14 out]
  n478 = call "qTCT.vi"() -> ()  [unwired: 2 in, 18 out]
  n479 = call "qTCV.vi"() -> ()  [unwired: 5 in, 15 out]
  n480 = call "TIM.vi"() -> ()  [unwired: 5 in, 15 out]
  n481 = call "qTIM.vi"() -> ()  [unwired: 2 in, 18 out]
  n482 = call "qTIO.vi"() -> ()  [unwired: 2 in, 18 out]
  n483 = call "qTMC.vi"() -> ()  [unwired: 2 in, 18 out]
  n484 = call "qTMP.vi"() -> ()  [unwired: 2 in, 18 out]
  n485 = call "qTNC.vi"() -> ()  [unwired: 2 in, 18 out]
  n486 = call "qTNR.vi"() -> ()  [unwired: 2 in, 18 out]
  n487 = call "qTPC.vi"() -> ()  [unwired: 2 in, 18 out]
  n488 = call "qTRC.vi"() -> ()  [unwired: 2 in, 18 out]
  n489 = call "TRO.vi"() -> ()  [unwired: 4 in, 16 out]
  n490 = call "qTRO.vi"() -> ()  [unwired: 4 in, 16 out]
  n491 = call "qTVI.vi"() -> ()  [unwired: 3 in, 17 out]
  n492 = call "UCL.vi"() -> ()  [unwired: 19 in, 1 out]
  n493 = call "qUCL.vi"() -> ()  [unwired: 18 in, 2 out]
  n494 = call "qVLS.vi"() -> ()  [unwired: 2 in, 18 out]
  n495 = call "qVST.vi"() -> ()  [unwired: 2 in, 18 out]
  n496 = call "WAA.vi"() -> ()  [unwired: 4 in, 16 out]
  n497 = call "WPA.vi"() -> ()  [unwired: 7 in, 13 out]
  n498 = call "TRI.vi"() -> ()  [unwired: 4 in, 16 out]
  n499 = call "qTRI.vi"() -> ()  [unwired: 4 in, 16 out]
  n500 = call "VLS.vi"() -> ()  [unwired: 4 in, 16 out]
  n501 = call "#9.vi"() -> ()  [unwired: 2 in, 18 out]
  n502 = call "DDL.vi"() -> ()  [unwired: 6 in, 14 out]
  n503 = call "qDDL.vi"() -> ()  [unwired: 5 in, 15 out]
  n504 = call "qDTL.vi"() -> ()  [unwired: 4 in, 16 out]
  n505 = call "qGWD.vi"() -> ()  [unwired: 6 in, 14 out]
  n506 = call "Send WG commands and wait for answers.vi"() -> ()  [unwired: 3 in, 17 out]
  n507 = call "SWT.vi"() -> ()  [unwired: 6 in, 14 out]
  n508 = call "qSWT.vi"() -> ()  [unwired: 4 in, 16 out]
  n509 = call "TGA.vi"() -> ()  [unwired: 5 in, 15 out]
  n510 = call "TGC.vi"() -> ()  [unwired: 3 in, 17 out]
  n511 = call "TGF.vi"() -> ()  [unwired: 3 in, 17 out]
  n512 = call "qTGL.vi"() -> ()  [unwired: 4 in, 16 out]
  n513 = call "TGS.vi"() -> ()  [unwired: 4 in, 16 out]
  n514 = call "TGT.vi"() -> ()  [unwired: 3 in, 17 out]
  n515 = call "qTGT.vi"() -> ()  [unwired: 2 in, 18 out]
  n516 = call "qTLT.vi"() -> ()  [unwired: 2 in, 18 out]
  n517 = call "TWC.vi"() -> ()  [unwired: 2 in, 18 out]
  n518 = call "qTWG.vi"() -> ()  [unwired: 2 in, 18 out]
  n519 = call "TWS.vi"() -> ()  [unwired: 5 in, 15 out]
  n520 = call "qTWS.vi"() -> ()  [unwired: 7 in, 13 out]
  n521 = call "WAV CFG.vi"() -> ()  [unwired: 5 in, 15 out]
  n522 = call "WAV.vi"() -> ()  [unwired: 20 in, 8 out]
  n523 = call "qWAV.vi"() -> ()  [unwired: 4 in, 16 out]
  n524 = call "WCL.vi"() -> ()  [unwired: 5 in, 15 out]
  n525 = call "WGC.vi"() -> ()  [unwired: 4 in, 16 out]
  n526 = call "qWGC.vi"() -> ()  [unwired: 5 in, 15 out]
  n527 = call "WGO.vi"() -> ()  [unwired: 4 in, 16 out]
  n528 = call "qWGO.vi"() -> ()  [unwired: 5 in, 15 out]
  n529 = call "WGR.vi"() -> ()  [unwired: 2 in, 18 out]
  n530 = call "WMS.vi"() -> ()  [unwired: 5 in, 15 out]
  n531 = call "qWMS.vi"() -> ()  [unwired: 5 in, 15 out]
  n532 = call "WOS.vi"() -> ()  [unwired: 5 in, 15 out]
  n533 = call "qWOS.vi"() -> ()  [unwired: 4 in, 16 out]
  n534 = call "WSL.vi"() -> ()  [unwired: 4 in, 16 out]
  n535 = call "qWSL.vi"() -> ()  [unwired: 4 in, 16 out]
  n536 = call "WTO.vi"() -> ()  [unwired: 6 in, 14 out]
  n537 = call "WTR.vi"() -> ()  [unwired: 5 in, 15 out]
  n538 = call "qWTR.vi"() -> ()  [unwired: 4 in, 16 out]
  n539 = call "qWGI.vi"() -> ()  [unwired: 5 in, 15 out]
  n540 = call "qWGN.vi"() -> ()  [unwired: 5 in, 15 out]
  n541 = call "qWGS.vi"() -> ()  [unwired: 5 in, 15 out]
  n542 = call "ConvertStatusRegisterToAxisStatus.vi"() -> ()  [unwired: 18 in, 2 out]
  n543 = call "ConvertStatusRegisterToSystemStatus.vi"() -> ()  [unwired: 18 in, 2 out]
  n544 = call "ConvertStatusRegistersToAxisStatusArray.vi"() -> ()  [unwired: 18 in, 2 out]
  n545 = call "ConvertStatusRegistersToSystemStatusArray.vi"() -> ()  [unwired: 18 in, 2 out]
  n546 = call "Analyse input string for terminal.vi"() -> ()  [unwired: 2 in, 18 out]
  n547 = call "Assign booleans from string to axes.vi"() -> ()  [unwired: 5 in, 15 out]
  n548 = call "Assign DRC values.vi"() -> ()  [unwired: 3 in, 17 out]
  n549 = call "Assign DRT values from string.vi"() -> ()  [unwired: 7 in, 13 out]
  n550 = call "Assign NaN for chosen axes.vi"() -> ()  [unwired: 4 in, 16 out]
  n551 = call "Assign SPA values from string to axes.vi"() -> ()  [unwired: 7 in, 13 out]
  n552 = call "Assign three values from string to axes.vi"() -> ()  [unwired: 3 in, 17 out]
  n553 = call "Assign values from string to axes.vi"() -> ()  [unwired: 6 in, 14 out]
  n554 = call "Axes_settled.vi"() -> ()  [unwired: 5 in, 15 out]
  n555 = call "Boolean array calculations.vi"() -> ()  [unwired: 4 in, 16 out]
  n556 = call "Build channel query command substring.vi"() -> ()  [unwired: 7 in, 13 out]
  n557 = call "Build command substring.vi"() -> ()  [unwired: 7 in, 13 out]
  n558 = call "Build qDIO query command substring.vi"() -> ()  [unwired: 6 in, 14 out]
  n559 = call "Build MVS command substring.vi"() -> ()  [unwired: 6 in, 14 out]
  n560 = call "Build num command substring.vi"() -> ()  [unwired: 3 in, 17 out]
  n561 = call "Build query command substring.vi"() -> ()  [unwired: 5 in, 15 out]
  n562 = call "Build qREL query command substring.vi"() -> ()  [unwired: 5 in, 15 out]
  n563 = call "Build SPA command substring.vi"() -> ()  [unwired: 10 in, 10 out]
  n564 = call "Build SPA query command substring.vi"() -> ()  [unwired: 5 in, 15 out]
  n565 = call "Build stringplusnum substring.vi"() -> ()  [unwired: 10 in, 10 out]
  n566 = call "Build WAV command substring.vi"() -> ()  [unwired: 19 in, 9 out]
  n567 = call "Commanded axes connected.vi"() -> ()  [unwired: 3 in, 17 out]
  n568 = call "Commanded stage name available.vi"() -> ()  [unwired: 3 in, 17 out]
  n569 = call "Convert error to warning.vi"() -> ()  [unwired: 2 in, 18 out]
  n570 = call "Convert num array to string.vi"() -> ()  [unwired: 2 in, 18 out]
  n571 = call "Convert num value to syntax selection.vi"() -> ()  [unwired: 1 in, 19 out]
  n572 = call "Count occurrences in string.vi"() -> ()  [unwired: 2 in, 18 out]
  n573 = call "Cut out additional spaces.vi"() -> ()  [unwired: 2 in, 18 out]
  n574 = call "Decode status bit.vi"() -> ()  [unwired: 2 in, 18 out]
  n575 = call "Define axes to command from boolean array.vi"() -> ()  [unwired: 4 in, 16 out]
  n576 = call "Define connected stages with dialog.vi"() -> ()  [unwired: 2 in, 18 out]
  n577 = call "Determine angular axis.vi"() -> ()  [unwired: 4 in, 16 out]
  n578 = call "GCSTranslateError.vi"() -> ()  [unwired: 1 in, 19 out]
  n579 = call "General wait for movement to stop.vi"() -> ()  [unwired: 8 in, 12 out]
  n580 = call "Get all axes.vi"() -> ()  [unwired: 1 in, 19 out]
  n581 = call "Get arrays without blanks.vi"() -> ()  [unwired: 3 in, 17 out]
  n582 = call "Get Controller Name from IDN.vi"() -> ()  [unwired: 2 in, 18 out]
  n583 = call "Get lines and values from string.vi"() -> ()  [unwired: 2 in, 18 out]
  n584 = call "Get lines from string.vi"() -> ()  [unwired: 3 in, 17 out]
  n585 = call "Split text segments from line.vi"() -> ()  [unwired: 19 in, 1 out]
  n586 = call "Get Slave Device Info.vi"() -> ()  [unwired: 2 in, 18 out]
  n587 = call "GCS3_Prepare_Motion_Error.vi"() -> ()  [unwired: 17 in, 3 out]
  n588 = call-poly "ConvertStatusRegister.vi"() -> ()  [unwired: 18 in, 2 out]
  n589 = call "Assign two values from string to axes.vi"() -> ()  [unwired: 3 in, 17 out]
  n590 = call "Build HIA command substring.vi"() -> ()  [unwired: 4 in, 16 out]
  n591 = call "Combine axes arrays.vi"() -> ()  [unwired: 2 in, 18 out]
  n592 = call "CST handler.vi"() -> ()  [unwired: 6 in, 14 out]
  n593 = call "Get string array size without blanks.vi"() -> ()  [unwired: 1 in, 19 out]
  n594 = call "Get total number of commanded axes.vi"() -> ()  [unwired: 2 in, 18 out]
  n595 = call "How often does string contain regular expression.vi"() -> ()  [unwired: 2 in, 18 out]
  n596 = call "HasMotionError.vi"() -> ()  [unwired: 18 in, 2 out]
  n597 = call "Increase array size.vi"() -> ()  [unwired: 3 in, 17 out]
  n598 = call "InMotion.vi"() -> ()  [unwired: 17 in, 3 out]
  n599 = call "IsControllerBusy.vi"() -> ()  [unwired: 18 in, 2 out]
  n600 = call-poly "Is command present in HLP answer.vi"() -> ()  [unwired: 5 in, 15 out]
  n601 = call "Longlasting one-axis command.vi"() -> ()  [unwired: 7 in, 13 out]
  n602 = call "Manual VMO.vi"() -> ()  [unwired: 6 in, 14 out]
  n603 = call "Move axes to their middle position.vi"() -> ()  [unwired: 5 in, 15 out]
  n604 = call "Multi Axis Query.vi"() -> ()  [unwired: 14 in, 2 out]
  n605 = call "Parse qKLS type answer by type.vi"() -> ()  [unwired: 3 in, 17 out]
  n606 = call "Parse qLOG Answer.vi"() -> ()  [unwired: 18 in, 2 out]
  n607 = call "Parse qUSG CMD Answer.vi"() -> ()  [unwired: 18 in, 2 out]
  n608 = call "Parse qUSG PAM Answer.vi"() -> ()  [unwired: 18 in, 2 out]
  n609 = call "Parse qUSG SYS Answer.vi"() -> ()  [unwired: 18 in, 2 out]
  n610 = call "ReadControllerInformation.vi"() -> ()  [unwired: 15 in, 5 out]
  n611 = call "Return single characters from string.vi"() -> ()  [unwired: 3 in, 17 out]
  n612 = call "Return space.vi"() -> ()  [unwired: 2 in, 18 out]
  n613 = call "Round with options.vi"() -> ()  [unwired: 4 in, 16 out]
  n614 = call "Select axis.vi"() -> ()  [unwired: 2 in, 18 out]
  n615 = call "Select values for chosen axes.vi"() -> ()  [unwired: 5 in, 15 out]
  n616 = call "Select with boolean array input.vi"() -> ()  [unwired: 4 in, 16 out]
  n617 = call "Selection to String array.vi"() -> ()  [unwired: 2 in, 18 out]
  n618 = call "Send string and wait for answer or timeout.vi"() -> ()  [unwired: 6 in, 14 out]
  n619 = call "Set RON and return RON status.vi"() -> ()  [unwired: 5 in, 15 out]
  n620 = call "Split multiple axes command.vi"() -> ()  [unwired: 9 in, 11 out]
  n621 = call "String with ASCII code conversion.vi"() -> ()  [unwired: 1 in, 19 out]
  n622 = call "Substract axes array subset from axes array.vi"() -> ()  [unwired: 2 in, 18 out]
  n623 = call "UnbundeBundle interface clusters for PI Terminal.vi"() -> ()  [unwired: 6 in, 14 out]
  n624 = call "Wait for answer 0 or 1 without polling.vi"() -> ()  [unwired: 5 in, 15 out]
  n625 = call "Wait for answer of longlasting command.vi"() -> ()  [unwired: 3 in, 17 out]
  n626 = call "Wait for axes to stop.vi"() -> ()  [unwired: 7 in, 13 out]
  n627 = call "Wait for controller ready.vi"() -> ()  [unwired: 4 in, 16 out]
  n628 = call "GCSArray_difference.vi"() -> ()  [unwired: 3 in, 17 out]
  n629 = call "GCSArray_header_read.vi"() -> ()  [unwired: 3 in, 17 out]
  n630 = call "GCSArray_import.vi"() -> ()  [unwired: 3 in, 17 out]
  n631 = call "GCSArray_intersection.vi"() -> ()  [unwired: 3 in, 17 out]
  n632 = call "GCSArray_regex_matches.vi"() -> ()  [unwired: 4 in, 16 out]
  n633 = call "GCSArray_regex_select.vi"() -> ()  [unwired: 4 in, 16 out]
  n634 = call "GCSArray_regex_string.vi"() -> ()  [unwired: 2 in, 18 out]
  n635 = call "GCSArray_valid.vi"() -> ()  [unwired: 4 in, 16 out]
  n636 = call "Parse_FRH_Type_String.vi"() -> ()  [unwired: 3 in, 17 out]
  n637 = call "Sep axes ini result in order.vi"() -> ()  [unwired: 2 in, 18 out]
  n638 = call "StopAllMotion.vi"() -> ()  [unwired: 19 in, 1 out]
